vi "CANOpen_Get Node ID from Name.vi"(11 "Node ID Name":string) -> (3 "Node ID":u8)   [LabVIEW 2013, in "CANOpen Addon Custom Device.lvlib"]
uses:
  CANOpen Addon Custom Device.lvlib
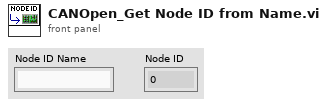
[diagram p1: front panel]
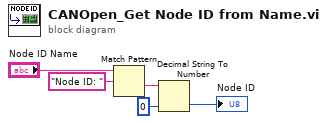
[diagram p0: block diagram]
diagram:
  n1 = Match Pattern(string="Node ID Name", regular expression="Node ID: ") -> (after substring=w4:string)  [unwired: 1 in, 3 out]
  n2 = Decimal String To Number(string=w4, default (0L)=u8 0 ("default (0 I32)")) -> (number=→"Node ID":u8)  [unwired: 1 in, 1 out]
